vi "draw_points.vi"(8 "XY Graph Ref In":refnum<vi>, 9 "Cycle":string(combo), 10 "T cluster":T2, 11 "P cluster":T3) -> (2 "XY Graph Ref Out":refnum<vi>, 3 "Table":string[][](array[string]))   [LabVIEW 2017]
panel:
  out "points array":T1(array[cluster])
  out "error out":errorcluster
  out "Application Directory 2":path
  out "Application Directory":path
  out "Points":dbl[][](array[numeric])
  out "P10":dbl
  out "XY Graph":cluster{dbl[], dbl[]}(graph)
  out "output cluster":cluster{dbl[], dbl[]}
  out "P11":dbl
  out "P5":dbl
  out "P4":dbl
  out "P3":dbl
  out "P2":dbl
  out "P1":dbl
  out "T11":dbl
  out "T10":dbl
  out "T9":dbl
  out "T8":dbl
  out "T7":dbl
  out "T6":dbl
  out "T5":dbl
  out "T4":dbl
  out "T3":dbl
  out "T2":dbl
  out "T1":dbl
  out "H Point 3":dbl
  out "Loop Iteration":i32
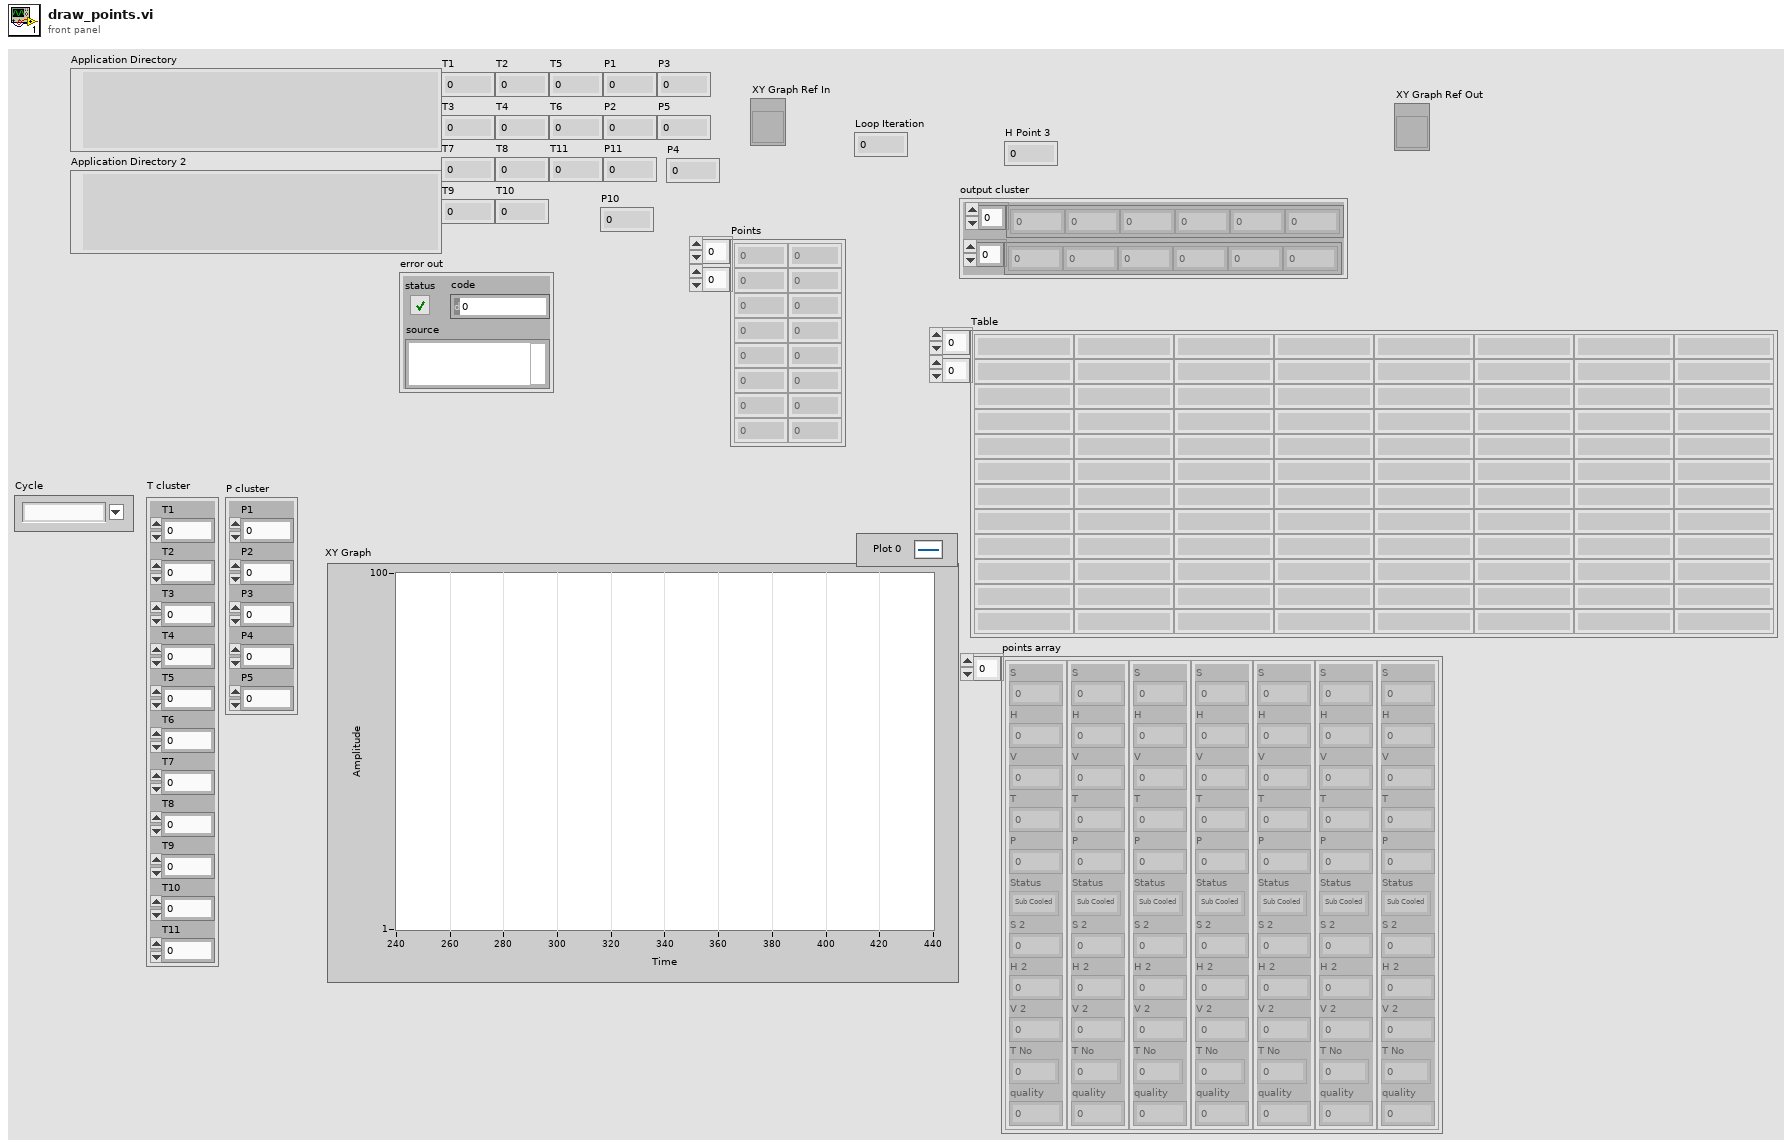
[diagram p1: front panel]
types:
  T1 = cluster{"S":dbl, "H":dbl, "V":dbl, "T":dbl, "P":dbl, "Status":enum16{"Sub Cooled", "Saturation", "Super Heated"}, "S 2":dbl, "H 2":dbl, "V 2":dbl, "T No":enum16{"0", "1", "2", "3", "4"}, "quality":dbl}[]
  T2 = cluster{"T1":dbl, "T2":dbl, "T3":dbl, "T4":dbl, "T5":dbl, "T6":dbl, "T7":dbl, "T8":dbl, "T9":dbl, "T10":dbl, "T11":dbl}
  T3 = cluster{"P1":dbl, "P2":dbl, "P3":dbl, "P4":dbl, "P5":dbl}
  T4 = cluster{"Name":string, "Color":u32, "Style":u8, "Point Style":u8, "Name Visible":bool, "Allow Drag":bool, "Annotation Mode":u32, "Plot":i32, "Index":i32, "Position":cluster{"X":dbl, "Y":dbl}, "X Scale":u32, "Y Scale":u32, "Show Arrow":bool, "Lock Name":bool, "Plot Area":i32, "Label Offset":cluster{"X":dbl, "Y":dbl}}
  T5 = cluster{"S":dbl, "H":dbl, "V":dbl, "T":dbl, "P":dbl, "Status":enum16{"Sub Cooled", "Saturation", "Super Heated"}, "S 2":dbl, "H 2":dbl, "V 2":dbl, "T No":enum16{"0", "1", "2", "3", "4"}, "quality":dbl}
  T6 = enum16{"Sub Cooled", "Saturation", "Super Heated"}
  T7 = typedef "LVAnnotationListTypeDef.ctl" = cluster{"Name":string, "Color":u32, "Style":u8, "Point Style":u8, "Name Visible":bool, "Allow Drag":bool, "Annotation Mode":u32, "Plot":i32, "Index":i32, "Position":cluster{"X":dbl, "Y":dbl}, "X Scale":u32, "Y Scale":u32, "Show Arrow":bool, "Lock Name":bool, "Plot Area":i32, "Label Offset":cluster{"X":dbl, "Y":dbl}}[]
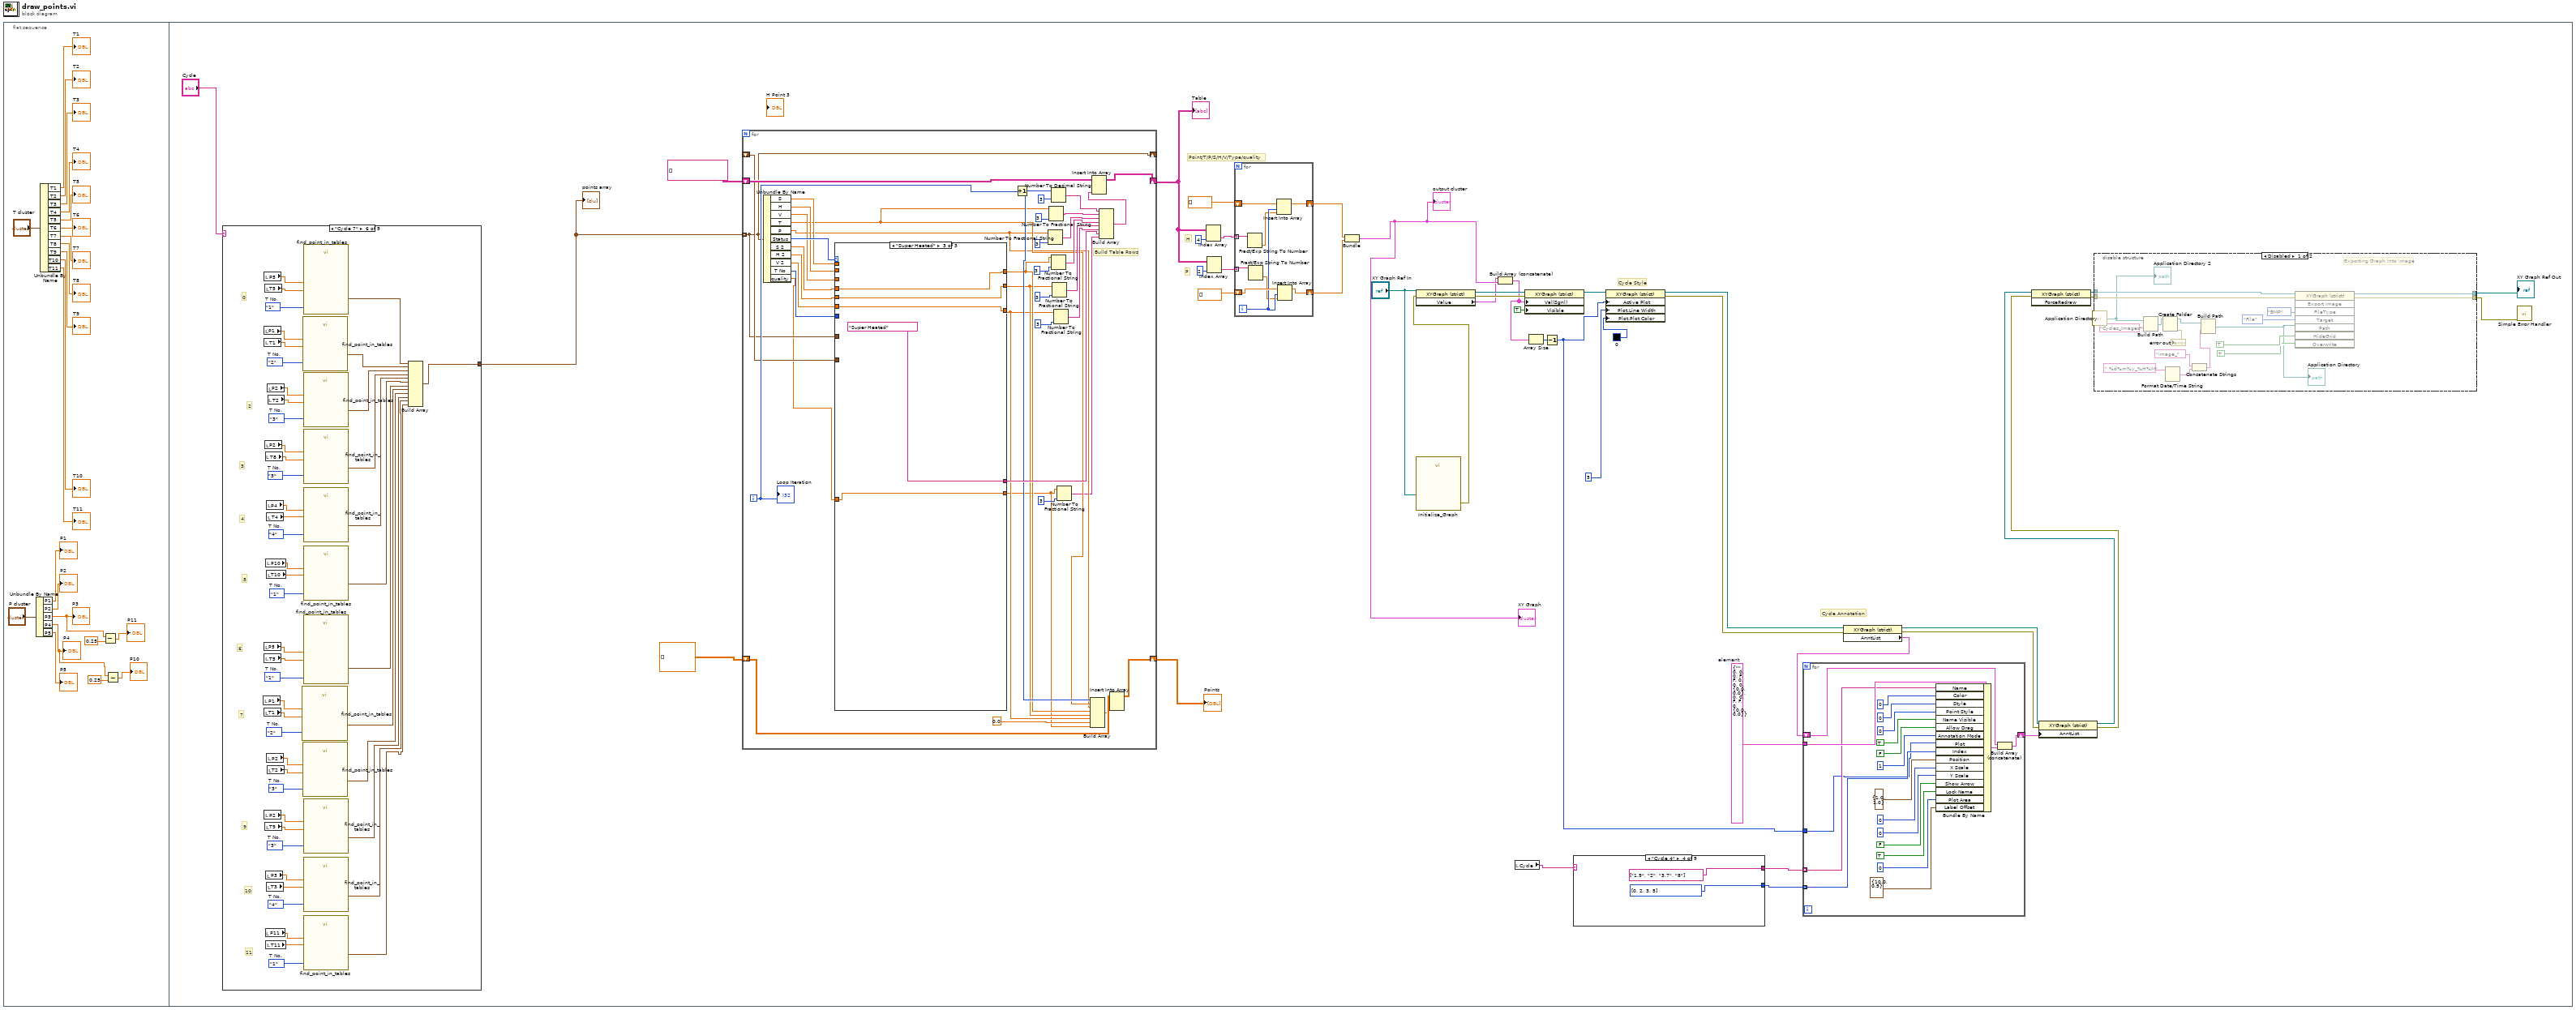
[diagram p0: block diagram]
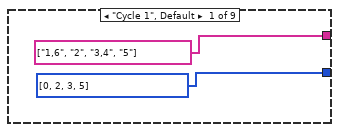
[diagram p3: hidden frame]
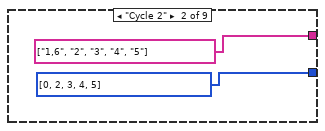
[diagram p4: hidden frame]
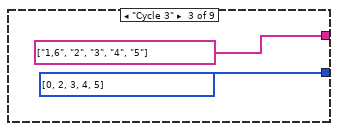
[diagram p5: hidden frame]
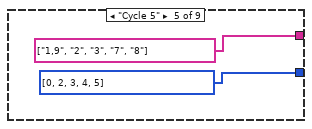
[diagram p6: hidden frame]
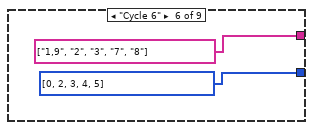
[diagram p7: hidden frame]
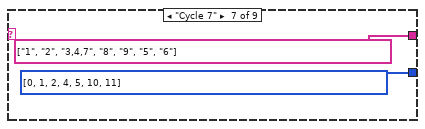
[diagram p8: hidden frame]
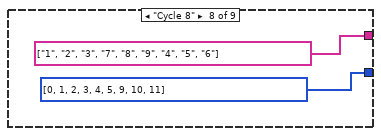
[diagram p9: hidden frame]
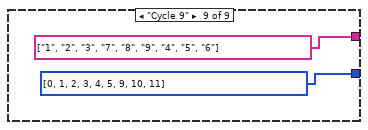
[diagram p10: hidden frame]
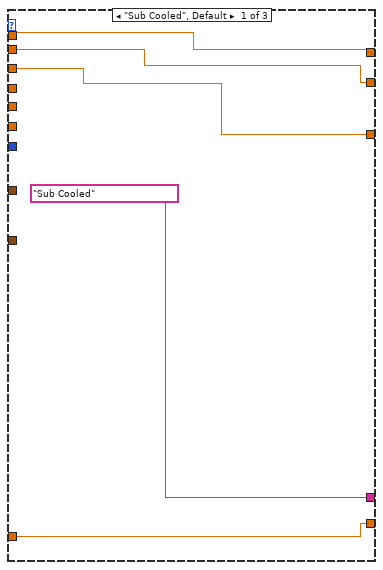
[diagram p11: hidden frame]
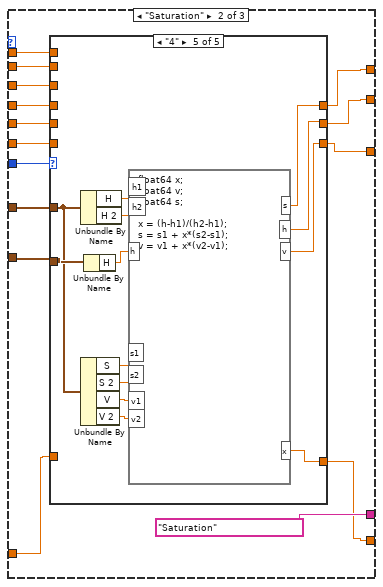
[diagram p12: hidden frame]
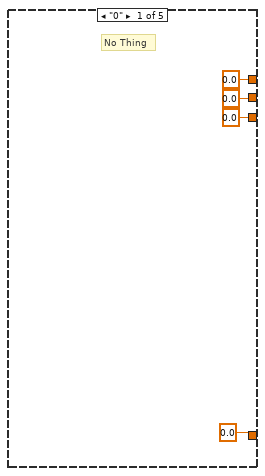
[diagram p13: hidden frame]
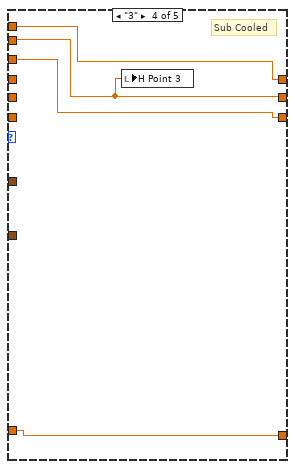
[diagram p16: hidden frame]
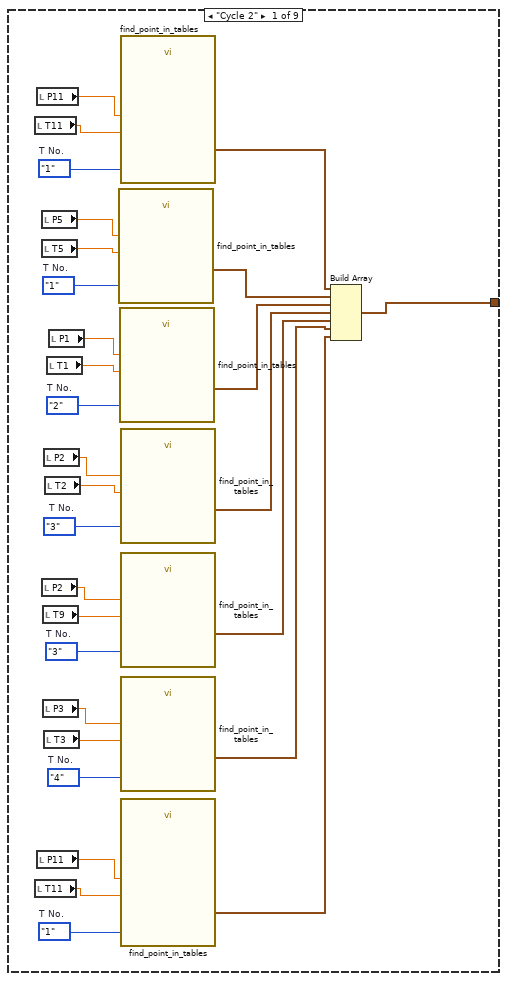
[diagram p17: hidden frame]
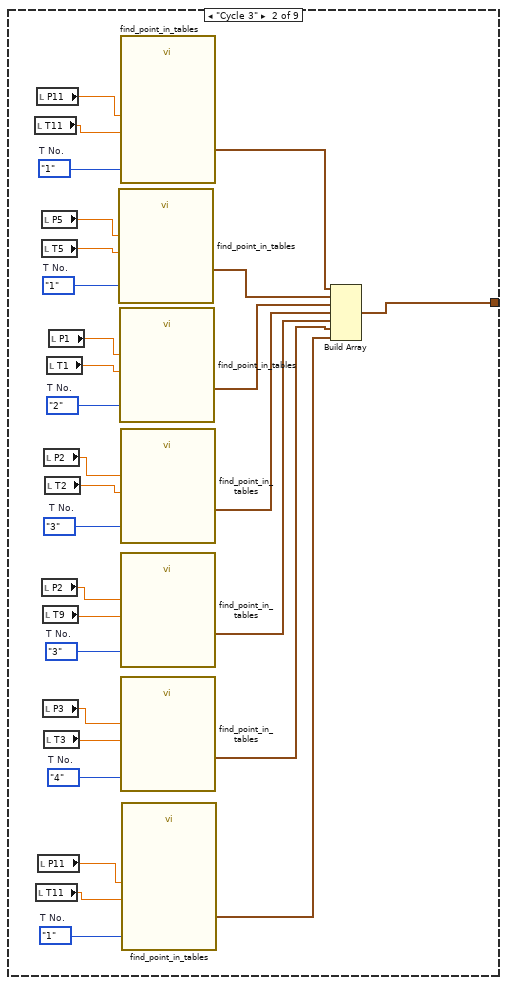
[diagram p18: hidden frame]
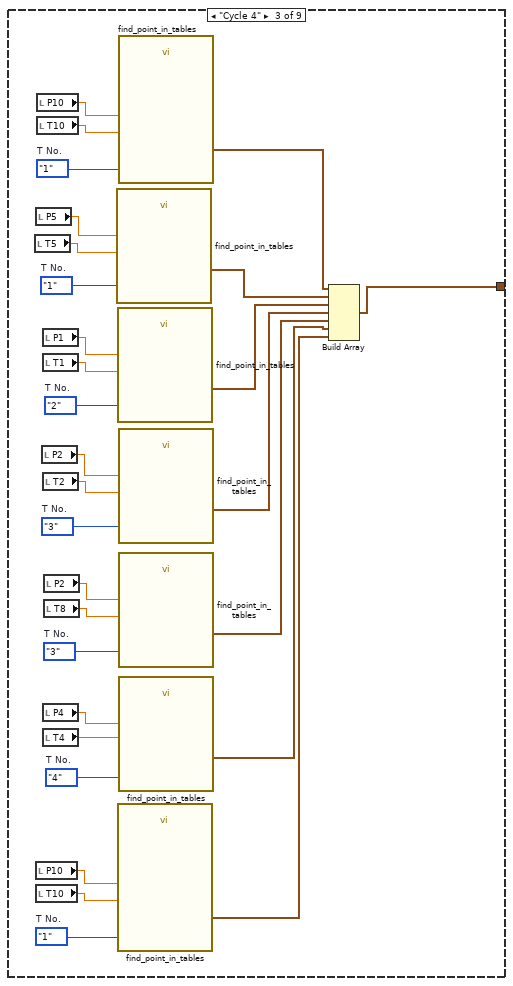
[diagram p19: hidden frame]
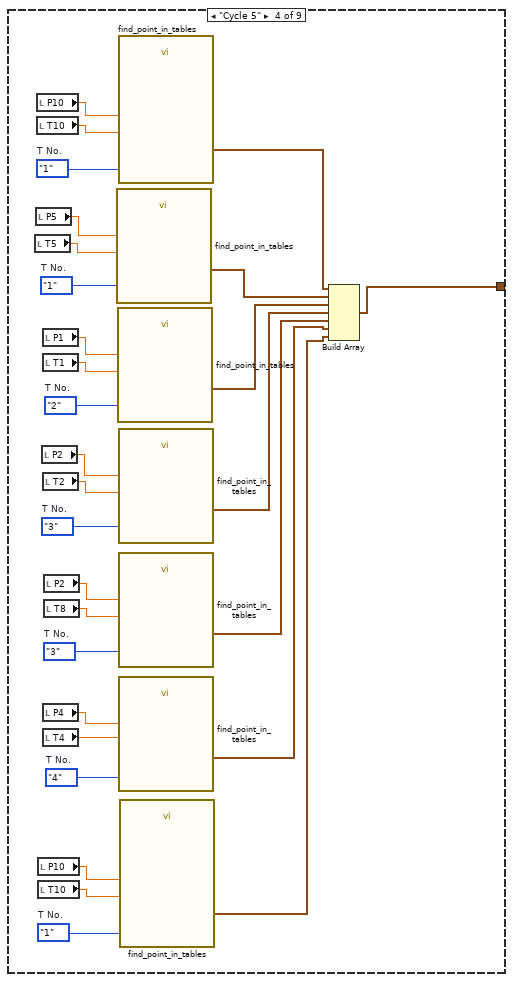
[diagram p20: hidden frame]
diagram:
  n1 = flat-sequence {
    frame #0 {
      n2 = Unbundle By Name("P cluster") -> ("P1"=→"P1":dbl, "P2"=→"P2":dbl, "P3"=w4:dbl, "P4"=w1:dbl, "P5"=→"P5":dbl)
      "P3" <- w4
      "P4" <- w1
      n3 = Unbundle By Name("T cluster") -> ("T1"=→"T1":dbl, "T2"=→"T2":dbl, "T3"=→"T3":dbl, "T4"=→"T4":dbl, "T5"=→"T5":dbl, "T6"=→"T6":dbl, "T7"=→"T7":dbl, "T8"=→"T8":dbl, "T9"=→"T9":dbl, "T10"=→"T10":dbl, "T11"=→"T11":dbl)
      n4 = Subtract(x=w4, y=0.25) -> (x-y=→"P11":dbl)
      n5 = Subtract(x=w1, y=0.25) -> (x-y=→"P10":dbl)
    }
    frame #1 {
      w41 = T4 {"Name"="", "Color"=0, "Style"=0, "Point Style"=0, "Name Visible"=FALSE, "Allow Drag"=FALSE, "Annotation Mode"=0, "Plot"=0, "Index"=0, "Position"={"X"=0.0, "Y"=0.0}, "X Scale"=0, "Y Scale"=0, "Show Arrow"=FALSE, "Lock Name"=FALSE, "Plot Area"=0, "Label Offset"={"X"=0.0, "Y"=0.0}}  # element
      # "Cycle Annotation"
      # "Cycle Style"
      # "H"
      # "P"
      # "Point/T/P/S/H/V/Type/quality"
      n6 = case shown="\"Cycle 7\"" "Cycle" {
        tunnel: [w232 w261 w302 w331 w360 w409 w458 w507 w540] -> w23
        frame "Cycle 2" {
          w229 = enum16{"0", "1", "2", "3", "4"}."1"  # T No.
          w245 = enum16{"0", "1", "2", "3", "4"}."4"  # T No.
          w246 = enum16{"0", "1", "2", "3", "4"}."3"  # T No.
          w247 = enum16{"0", "1", "2", "3", "4"}."3"  # T No.
          w248 = enum16{"0", "1", "2", "3", "4"}."2"  # T No.
          w249 = enum16{"0", "1", "2", "3", "4"}."1"  # T No.
          w250 = enum16{"0", "1", "2", "3", "4"}."1"  # T No.
          n7 = local read "T11"() -> (w243:dbl)
          n8 = local read "T11"() -> (w231:dbl)
          n9 = local read "P11"() -> (w244:dbl)
          n10 = local read "P11"() -> (w230:dbl)
          n11 = local read "P5"() -> (w242:dbl)
          n12 = local read "T5"() -> (w241:dbl)
          n13 = local read "P2"() -> (w236:dbl)
          n14 = local read "T9"() -> (w235:dbl)
          n15 = local read "P3"() -> (w234:dbl)
          n16 = local read "P2"() -> (w238:dbl)
          n17 = local read "T3"() -> (w233:dbl)
          n18 = local read "T2"() -> (w237:dbl)
          n19 = local read "T1"() -> (w239:dbl)
          n20 = local read "P1"() -> (w240:dbl)
          n21 = call "find_point_in_tables.vi"("T No."=w249, "T Search"=w241, "P Search"=w242) -> ("Point"=w254:T5)  [unwired: 7 in]
          n22 = call "find_point_in_tables.vi"("T No."=w248, "T Search"=w239, "P Search"=w240) -> ("Point"=w255:T5)  [unwired: 7 in]
          n23 = call "find_point_in_tables.vi"("T No."=w250, "T Search"=w243, "P Search"=w244) -> ("Point"=w253:T5)  [unwired: 7 in]
          n24 = call "find_point_in_tables.vi"("T No."=w247, "T Search"=w237, "P Search"=w238) -> ("Point"=w256:T5)  [unwired: 7 in]
          n25 = call "find_point_in_tables.vi"("T No."=w246, "T Search"=w235, "P Search"=w236) -> ("Point"=w252:T5)  [unwired: 7 in]
          n26 = call "find_point_in_tables.vi"("T No."=w245, "T Search"=w233, "P Search"=w234) -> ("Point"=w251:T5)  [unwired: 7 in]
          n27 = call "find_point_in_tables.vi"("T No."=w229, "T Search"=w231, "P Search"=w230) -> ("Point"=w228:T5)  [unwired: 7 in]
          n28 = Build Array(w253, w254, w255, w256, w252, w251, w228) -> (w232:T1)
        }
        frame "Cycle 3" {
          w258 = enum16{"0", "1", "2", "3", "4"}."1"  # T No.
          w274 = enum16{"0", "1", "2", "3", "4"}."4"  # T No.
          w275 = enum16{"0", "1", "2", "3", "4"}."3"  # T No.
          w276 = enum16{"0", "1", "2", "3", "4"}."3"  # T No.
          w277 = enum16{"0", "1", "2", "3", "4"}."2"  # T No.
          w278 = enum16{"0", "1", "2", "3", "4"}."1"  # T No.
          w279 = enum16{"0", "1", "2", "3", "4"}."1"  # T No.
          n29 = local read "T11"() -> (w272:dbl)
          n30 = local read "T11"() -> (w260:dbl)
          n31 = local read "P11"() -> (w273:dbl)
          n32 = local read "P11"() -> (w259:dbl)
          n33 = local read "P5"() -> (w271:dbl)
          n34 = local read "T5"() -> (w270:dbl)
          n35 = local read "P2"() -> (w265:dbl)
          n36 = local read "T9"() -> (w264:dbl)
          n37 = local read "P3"() -> (w263:dbl)
          n38 = local read "P2"() -> (w267:dbl)
          n39 = local read "T3"() -> (w262:dbl)
          n40 = local read "T2"() -> (w266:dbl)
          n41 = local read "T1"() -> (w268:dbl)
          n42 = local read "P1"() -> (w269:dbl)
          n43 = call "find_point_in_tables.vi"("T No."=w278, "T Search"=w270, "P Search"=w271) -> ("Point"=w283:T5)  [unwired: 7 in]
          n44 = call "find_point_in_tables.vi"("T No."=w277, "T Search"=w268, "P Search"=w269) -> ("Point"=w284:T5)  [unwired: 7 in]
          n45 = call "find_point_in_tables.vi"("T No."=w279, "T Search"=w272, "P Search"=w273) -> ("Point"=w282:T5)  [unwired: 7 in]
          n46 = call "find_point_in_tables.vi"("T No."=w276, "T Search"=w266, "P Search"=w267) -> ("Point"=w285:T5)  [unwired: 7 in]
          n47 = call "find_point_in_tables.vi"("T No."=w275, "T Search"=w264, "P Search"=w265) -> ("Point"=w281:T5)  [unwired: 7 in]
          n48 = call "find_point_in_tables.vi"("T No."=w274, "T Search"=w262, "P Search"=w263) -> ("Point"=w280:T5)  [unwired: 7 in]
          n49 = call "find_point_in_tables.vi"("T No."=w258, "T Search"=w260, "P Search"=w259) -> ("Point"=w257:T5)  [unwired: 7 in]
          n50 = Build Array(w282, w283, w284, w285, w281, w280, w257) -> (w261:T1)
        }
        frame "Cycle 4" {
          w287 = enum16{"0", "1", "2", "3", "4"}."1"  # T No.
          w303 = enum16{"0", "1", "2", "3", "4"}."4"  # T No.
          w304 = enum16{"0", "1", "2", "3", "4"}."3"  # T No.
          w305 = enum16{"0", "1", "2", "3", "4"}."3"  # T No.
          w306 = enum16{"0", "1", "2", "3", "4"}."2"  # T No.
          w307 = enum16{"0", "1", "2", "3", "4"}."1"  # T No.
          w308 = enum16{"0", "1", "2", "3", "4"}."1"  # T No.
          n51 = local read "T5"() -> (w298:dbl)
          n52 = local read "P5"() -> (w299:dbl)
          n53 = local read "P10"() -> (w289:dbl)
          n54 = local read "T10"() -> (w288:dbl)
          n55 = local read "P10"() -> (w300:dbl)
          n56 = local read "T10"() -> (w301:dbl)
          n57 = local read "P2"() -> (w295:dbl)
          n58 = local read "P1"() -> (w297:dbl)
          n59 = local read "T1"() -> (w296:dbl)
          n60 = local read "T2"() -> (w294:dbl)
          n61 = local read "P4"() -> (w291:dbl)
          n62 = local read "T4"() -> (w290:dbl)
          n63 = local read "P2"() -> (w293:dbl)
          n64 = local read "T8"() -> (w292:dbl)
          n65 = call "find_point_in_tables.vi"("T No."=w307, "T Search"=w298, "P Search"=w299) -> ("Point"=w312:T5)  [unwired: 7 in]
          n66 = call "find_point_in_tables.vi"("T No."=w306, "T Search"=w296, "P Search"=w297) -> ("Point"=w313:T5)  [unwired: 7 in]
          n67 = call "find_point_in_tables.vi"("T No."=w287, "T Search"=w288, "P Search"=w289) -> ("Point"=w286:T5)  [unwired: 7 in]
          n68 = call "find_point_in_tables.vi"("T No."=w308, "T Search"=w301, "P Search"=w300) -> ("Point"=w311:T5)  [unwired: 7 in]
          n69 = call "find_point_in_tables.vi"("T No."=w305, "T Search"=w294, "P Search"=w295) -> ("Point"=w314:T5)  [unwired: 7 in]
          n70 = call "find_point_in_tables.vi"("T No."=w304, "T Search"=w292, "P Search"=w293) -> ("Point"=w310:T5)  [unwired: 7 in]
          n71 = call "find_point_in_tables.vi"("T No."=w303, "T Search"=w290, "P Search"=w291) -> ("Point"=w309:T5)  [unwired: 7 in]
          n72 = Build Array(w311, w312, w313, w314, w310, w309, w286) -> (w302:T1)
        }
        frame "Cycle 5" {
          w316 = enum16{"0", "1", "2", "3", "4"}."1"  # T No.
          w332 = enum16{"0", "1", "2", "3", "4"}."4"  # T No.
          w333 = enum16{"0", "1", "2", "3", "4"}."3"  # T No.
          w334 = enum16{"0", "1", "2", "3", "4"}."3"  # T No.
          w335 = enum16{"0", "1", "2", "3", "4"}."2"  # T No.
          w336 = enum16{"0", "1", "2", "3", "4"}."1"  # T No.
          w337 = enum16{"0", "1", "2", "3", "4"}."1"  # T No.
          n73 = local read "T5"() -> (w327:dbl)
          n74 = local read "P5"() -> (w328:dbl)
          n75 = local read "P10"() -> (w329:dbl)
          n76 = local read "T10"() -> (w330:dbl)
          n77 = local read "P10"() -> (w318:dbl)
          n78 = local read "T10"() -> (w317:dbl)
          n79 = local read "P2"() -> (w324:dbl)
          n80 = local read "P1"() -> (w326:dbl)
          n81 = local read "T1"() -> (w325:dbl)
          n82 = local read "T2"() -> (w323:dbl)
          n83 = local read "P4"() -> (w320:dbl)
          n84 = local read "T4"() -> (w319:dbl)
          n85 = local read "P2"() -> (w322:dbl)
          n86 = local read "T8"() -> (w321:dbl)
          n87 = call "find_point_in_tables.vi"("T No."=w336, "T Search"=w327, "P Search"=w328) -> ("Point"=w341:T5)  [unwired: 7 in]
          n88 = call "find_point_in_tables.vi"("T No."=w335, "T Search"=w325, "P Search"=w326) -> ("Point"=w342:T5)  [unwired: 7 in]
          n89 = call "find_point_in_tables.vi"("T No."=w337, "T Search"=w330, "P Search"=w329) -> ("Point"=w340:T5)  [unwired: 7 in]
          n90 = call "find_point_in_tables.vi"("T No."=w334, "T Search"=w323, "P Search"=w324) -> ("Point"=w343:T5)  [unwired: 7 in]
          n91 = call "find_point_in_tables.vi"("T No."=w333, "T Search"=w321, "P Search"=w322) -> ("Point"=w339:T5)  [unwired: 7 in]
          n92 = call "find_point_in_tables.vi"("T No."=w332, "T Search"=w319, "P Search"=w320) -> ("Point"=w338:T5)  [unwired: 7 in]
          n93 = call "find_point_in_tables.vi"("T No."=w316, "T Search"=w317, "P Search"=w318) -> ("Point"=w315:T5)  [unwired: 7 in]
          n94 = Build Array(w340, w341, w342, w343, w339, w338, w315) -> (w331:T1)
        }
        frame "Cycle 6" {
          w345 = enum16{"0", "1", "2", "3", "4"}."1"  # T No.
          w361 = enum16{"0", "1", "2", "3", "4"}."4"  # T No.
          w362 = enum16{"0", "1", "2", "3", "4"}."3"  # T No.
          w363 = enum16{"0", "1", "2", "3", "4"}."3"  # T No.
          w364 = enum16{"0", "1", "2", "3", "4"}."2"  # T No.
          w365 = enum16{"0", "1", "2", "3", "4"}."1"  # T No.
          w366 = enum16{"0", "1", "2", "3", "4"}."1"  # T No.
          n95 = local read "T5"() -> (w356:dbl)
          n96 = local read "P5"() -> (w357:dbl)
          n97 = local read "P10"() -> (w358:dbl)
          n98 = local read "T10"() -> (w359:dbl)
          n99 = local read "P10"() -> (w347:dbl)
          n100 = local read "T10"() -> (w346:dbl)
          n101 = local read "P2"() -> (w353:dbl)
          n102 = local read "P1"() -> (w355:dbl)
          n103 = local read "T1"() -> (w354:dbl)
          n104 = local read "T2"() -> (w352:dbl)
          n105 = local read "P4"() -> (w349:dbl)
          n106 = local read "T4"() -> (w348:dbl)
          n107 = local read "P2"() -> (w351:dbl)
          n108 = local read "T8"() -> (w350:dbl)
          n109 = call "find_point_in_tables.vi"("T No."=w365, "T Search"=w356, "P Search"=w357) -> ("Point"=w370:T5)  [unwired: 7 in]
          n110 = call "find_point_in_tables.vi"("T No."=w364, "T Search"=w354, "P Search"=w355) -> ("Point"=w371:T5)  [unwired: 7 in]
          n111 = call "find_point_in_tables.vi"("T No."=w366, "T Search"=w359, "P Search"=w358) -> ("Point"=w369:T5)  [unwired: 7 in]
          n112 = call "find_point_in_tables.vi"("T No."=w363, "T Search"=w352, "P Search"=w353) -> ("Point"=w372:T5)  [unwired: 7 in]
          n113 = call "find_point_in_tables.vi"("T No."=w362, "T Search"=w350, "P Search"=w351) -> ("Point"=w368:T5)  [unwired: 7 in]
          n114 = call "find_point_in_tables.vi"("T No."=w361, "T Search"=w348, "P Search"=w349) -> ("Point"=w367:T5)  [unwired: 7 in]
          n115 = call "find_point_in_tables.vi"("T No."=w345, "T Search"=w346, "P Search"=w347) -> ("Point"=w344:T5)  [unwired: 7 in]
          n116 = Build Array(w369, w370, w371, w372, w368, w367, w344) -> (w360:T1)
        }
        frame "Cycle 7" {
          w384 = enum16{"0", "1", "2", "3", "4"}."1"  # T No.
          w383 = enum16{"0", "1", "2", "3", "4"}."4"  # T No.
          w382 = enum16{"0", "1", "2", "3", "4"}."3"  # T No.
          w381 = enum16{"0", "1", "2", "3", "4"}."3"  # T No.
          w380 = enum16{"0", "1", "2", "3", "4"}."2"  # T No.
          w379 = enum16{"0", "1", "2", "3", "4"}."1"  # T No.
          w410 = enum16{"0", "1", "2", "3", "4"}."1"  # T No.
          w411 = enum16{"0", "1", "2", "3", "4"}."4"  # T No.
          w412 = enum16{"0", "1", "2", "3", "4"}."3"  # T No.
          w413 = enum16{"0", "1", "2", "3", "4"}."3"  # T No.
          w414 = enum16{"0", "1", "2", "3", "4"}."2"  # T No.
          w415 = enum16{"0", "1", "2", "3", "4"}."1"  # T No.
          # "11"
          # "10"
          # "9"
          # "8"
          # "7"
          # "6"
          # "5"
          # "4"
          # "3"
          # "2"
          # "1"
          # "0"
          n117 = local read "P1"() -> (w387:dbl)
          n118 = local read "P1"() -> (w406:dbl)
          n119 = local read "P5"() -> (w385:dbl)
          n120 = local read "T1"() -> (w388:dbl)
          n121 = local read "P5"() -> (w408:dbl)
          n122 = local read "T1"() -> (w405:dbl)
          n123 = local read "T5"() -> (w386:dbl)
          n124 = local read "P2"() -> (w391:dbl)
          n125 = local read "T5"() -> (w407:dbl)
          n126 = local read "P2"() -> (w402:dbl)
          n127 = local read "T9"() -> (w392:dbl)
          n128 = local read "T8"() -> (w401:dbl)
          n129 = local read "P11"() -> (w395:dbl)
          n130 = local read "P10"() -> (w398:dbl)
          n131 = local read "P3"() -> (w393:dbl)
          n132 = local read "T11"() -> (w396:dbl)
          n133 = local read "P4"() -> (w400:dbl)
          n134 = local read "T10"() -> (w397:dbl)
          n135 = local read "T3"() -> (w394:dbl)
          n136 = local read "T4"() -> (w399:dbl)
          n137 = local read "P2"() -> (w389:dbl)
          n138 = local read "P2"() -> (w404:dbl)
          n139 = local read "T2"() -> (w390:dbl)
          n140 = local read "T2"() -> (w403:dbl)
          n141 = call "find_point_in_tables.vi"("T No."=w380, "T Search"=w388, "P Search"=w387) -> ("Point"=w377:T5)  [unwired: 7 in]
          n142 = call "find_point_in_tables.vi"("T No."=w414, "T Search"=w405, "P Search"=w406) -> ("Point"=w419:T5)  [unwired: 7 in]
          n143 = call "find_point_in_tables.vi"("T No."=w381, "T Search"=w390, "P Search"=w389) -> ("Point"=w376:T5)  [unwired: 7 in]
          n144 = call "find_point_in_tables.vi"("T No."=w413, "T Search"=w403, "P Search"=w404) -> ("Point"=w420:T5)  [unwired: 7 in]
          n145 = call "find_point_in_tables.vi"("T No."=w379, "T Search"=w386, "P Search"=w385) -> ("Point"=w378:T5)  [unwired: 7 in]
          n146 = call "find_point_in_tables.vi"("T No."=w382, "T Search"=w392, "P Search"=w391) -> ("Point"=w375:T5)  [unwired: 7 in]
          n147 = call "find_point_in_tables.vi"("T No."=w383, "T Search"=w394, "P Search"=w393) -> ("Point"=w374:T5)  [unwired: 7 in]
          n148 = call "find_point_in_tables.vi"("T No."=w384, "T Search"=w396, "P Search"=w395) -> ("Point"=w373:T5)  [unwired: 7 in]
          n149 = call "find_point_in_tables.vi"("T No."=w415, "T Search"=w407, "P Search"=w408) -> ("Point"=w418:T5)  [unwired: 7 in]
          n150 = call "find_point_in_tables.vi"("T No."=w412, "T Search"=w401, "P Search"=w402) -> ("Point"=w421:T5)  [unwired: 7 in]
          n151 = call "find_point_in_tables.vi"("T No."=w411, "T Search"=w399, "P Search"=w400) -> ("Point"=w417:T5)  [unwired: 7 in]
          n152 = call "find_point_in_tables.vi"("T No."=w410, "T Search"=w397, "P Search"=w398) -> ("Point"=w416:T5)  [unwired: 7 in]
          n153 = Build Array(w418, w419, w420, w421, w417, w416, w378, w377, w376, w375, w374, w373) -> (w409:T1)
        }
        frame "Cycle 8" {
          w433 = enum16{"0", "1", "2", "3", "4"}."1"  # T No.
          w432 = enum16{"0", "1", "2", "3", "4"}."4"  # T No.
          w431 = enum16{"0", "1", "2", "3", "4"}."3"  # T No.
          w430 = enum16{"0", "1", "2", "3", "4"}."3"  # T No.
          w429 = enum16{"0", "1", "2", "3", "4"}."2"  # T No.
          w428 = enum16{"0", "1", "2", "3", "4"}."1"  # T No.
          w459 = enum16{"0", "1", "2", "3", "4"}."1"  # T No.
          w460 = enum16{"0", "1", "2", "3", "4"}."4"  # T No.
          w461 = enum16{"0", "1", "2", "3", "4"}."3"  # T No.
          w462 = enum16{"0", "1", "2", "3", "4"}."3"  # T No.
          w463 = enum16{"0", "1", "2", "3", "4"}."2"  # T No.
          w464 = enum16{"0", "1", "2", "3", "4"}."1"  # T No.
          n154 = local read "P1"() -> (w436:dbl)
          n155 = local read "P1"() -> (w455:dbl)
          n156 = local read "P5"() -> (w434:dbl)
          n157 = local read "T1"() -> (w437:dbl)
          n158 = local read "P5"() -> (w457:dbl)
          n159 = local read "T1"() -> (w454:dbl)
          n160 = local read "T5"() -> (w435:dbl)
          n161 = local read "P2"() -> (w440:dbl)
          n162 = local read "T5"() -> (w456:dbl)
          n163 = local read "P2"() -> (w451:dbl)
          n164 = local read "T9"() -> (w441:dbl)
          n165 = local read "T8"() -> (w450:dbl)
          n166 = local read "P11"() -> (w444:dbl)
          n167 = local read "P10"() -> (w447:dbl)
          n168 = local read "P3"() -> (w442:dbl)
          n169 = local read "T11"() -> (w445:dbl)
          n170 = local read "P4"() -> (w449:dbl)
          n171 = local read "T10"() -> (w446:dbl)
          n172 = local read "T3"() -> (w443:dbl)
          n173 = local read "T4"() -> (w448:dbl)
          n174 = local read "T2"() -> (w438:dbl)
          n175 = local read "P2"() -> (w453:dbl)
          n176 = local read "P2"() -> (w439:dbl)
          n177 = local read "T2"() -> (w452:dbl)
          n178 = call "find_point_in_tables.vi"("T No."=w429, "T Search"=w437, "P Search"=w436) -> ("Point"=w426:T5)  [unwired: 7 in]
          n179 = call "find_point_in_tables.vi"("T No."=w463, "T Search"=w454, "P Search"=w455) -> ("Point"=w468:T5)  [unwired: 7 in]
          n180 = call "find_point_in_tables.vi"("T No."=w430, "T Search"=w439, "P Search"=w438) -> ("Point"=w425:T5)  [unwired: 7 in]
          n181 = call "find_point_in_tables.vi"("T No."=w462, "T Search"=w452, "P Search"=w453) -> ("Point"=w469:T5)  [unwired: 7 in]
          n182 = call "find_point_in_tables.vi"("T No."=w428, "T Search"=w435, "P Search"=w434) -> ("Point"=w427:T5)  [unwired: 7 in]
          n183 = call "find_point_in_tables.vi"("T No."=w431, "T Search"=w441, "P Search"=w440) -> ("Point"=w424:T5)  [unwired: 7 in]
          n184 = call "find_point_in_tables.vi"("T No."=w432, "T Search"=w443, "P Search"=w442) -> ("Point"=w423:T5)  [unwired: 7 in]
          n185 = call "find_point_in_tables.vi"("T No."=w433, "T Search"=w445, "P Search"=w444) -> ("Point"=w422:T5)  [unwired: 7 in]
          n186 = call "find_point_in_tables.vi"("T No."=w464, "T Search"=w456, "P Search"=w457) -> ("Point"=w467:T5)  [unwired: 7 in]
          n187 = call "find_point_in_tables.vi"("T No."=w461, "T Search"=w450, "P Search"=w451) -> ("Point"=w470:T5)  [unwired: 7 in]
          n188 = call "find_point_in_tables.vi"("T No."=w460, "T Search"=w448, "P Search"=w449) -> ("Point"=w466:T5)  [unwired: 7 in]
          n189 = call "find_point_in_tables.vi"("T No."=w459, "T Search"=w446, "P Search"=w447) -> ("Point"=w465:T5)  [unwired: 7 in]
          n190 = Build Array(w467, w468, w469, w470, w466, w465, w427, w426, w425, w424, w423, w422) -> (w458:T1)
        }
        frame "Cycle 9" {
          w482 = enum16{"0", "1", "2", "3", "4"}."1"  # T No.
          w481 = enum16{"0", "1", "2", "3", "4"}."4"  # T No.
          w480 = enum16{"0", "1", "2", "3", "4"}."3"  # T No.
          w479 = enum16{"0", "1", "2", "3", "4"}."3"  # T No.
          w478 = enum16{"0", "1", "2", "3", "4"}."2"  # T No.
          w477 = enum16{"0", "1", "2", "3", "4"}."1"  # T No.
          w508 = enum16{"0", "1", "2", "3", "4"}."1"  # T No.
          w509 = enum16{"0", "1", "2", "3", "4"}."4"  # T No.
          w510 = enum16{"0", "1", "2", "3", "4"}."3"  # T No.
          w511 = enum16{"0", "1", "2", "3", "4"}."3"  # T No.
          w512 = enum16{"0", "1", "2", "3", "4"}."2"  # T No.
          w513 = enum16{"0", "1", "2", "3", "4"}."1"  # T No.
          n191 = local read "P1"() -> (w485:dbl)
          n192 = local read "P1"() -> (w504:dbl)
          n193 = local read "P5"() -> (w483:dbl)
          n194 = local read "T1"() -> (w486:dbl)
          n195 = local read "P5"() -> (w506:dbl)
          n196 = local read "T1"() -> (w503:dbl)
          n197 = local read "T5"() -> (w484:dbl)
          n198 = local read "P2"() -> (w489:dbl)
          n199 = local read "T5"() -> (w505:dbl)
          n200 = local read "P2"() -> (w500:dbl)
          n201 = local read "T9"() -> (w490:dbl)
          n202 = local read "T8"() -> (w499:dbl)
          n203 = local read "P11"() -> (w493:dbl)
          n204 = local read "P10"() -> (w496:dbl)
          n205 = local read "P3"() -> (w491:dbl)
          n206 = local read "T11"() -> (w494:dbl)
          n207 = local read "P4"() -> (w498:dbl)
          n208 = local read "T10"() -> (w495:dbl)
          n209 = local read "T3"() -> (w492:dbl)
          n210 = local read "T4"() -> (w497:dbl)
          n211 = local read "T2"() -> (w487:dbl)
          n212 = local read "P2"() -> (w502:dbl)
          n213 = local read "P2"() -> (w488:dbl)
          n214 = local read "T2"() -> (w501:dbl)
          n215 = call "find_point_in_tables.vi"("T No."=w478, "T Search"=w486, "P Search"=w485) -> ("Point"=w475:T5)  [unwired: 7 in]
          n216 = call "find_point_in_tables.vi"("T No."=w512, "T Search"=w503, "P Search"=w504) -> ("Point"=w517:T5)  [unwired: 7 in]
          n217 = call "find_point_in_tables.vi"("T No."=w479, "T Search"=w488, "P Search"=w487) -> ("Point"=w474:T5)  [unwired: 7 in]
          n218 = call "find_point_in_tables.vi"("T No."=w511, "T Search"=w501, "P Search"=w502) -> ("Point"=w518:T5)  [unwired: 7 in]
          n219 = call "find_point_in_tables.vi"("T No."=w477, "T Search"=w484, "P Search"=w483) -> ("Point"=w476:T5)  [unwired: 7 in]
          n220 = call "find_point_in_tables.vi"("T No."=w480, "T Search"=w490, "P Search"=w489) -> ("Point"=w473:T5)  [unwired: 7 in]
          n221 = call "find_point_in_tables.vi"("T No."=w481, "T Search"=w492, "P Search"=w491) -> ("Point"=w472:T5)  [unwired: 7 in]
          n222 = call "find_point_in_tables.vi"("T No."=w482, "T Search"=w494, "P Search"=w493) -> ("Point"=w471:T5)  [unwired: 7 in]
          n223 = call "find_point_in_tables.vi"("T No."=w513, "T Search"=w505, "P Search"=w506) -> ("Point"=w516:T5)  [unwired: 7 in]
          n224 = call "find_point_in_tables.vi"("T No."=w510, "T Search"=w499, "P Search"=w500) -> ("Point"=w519:T5)  [unwired: 7 in]
          n225 = call "find_point_in_tables.vi"("T No."=w509, "T Search"=w497, "P Search"=w498) -> ("Point"=w515:T5)  [unwired: 7 in]
          n226 = call "find_point_in_tables.vi"("T No."=w508, "T Search"=w495, "P Search"=w496) -> ("Point"=w514:T5)  [unwired: 7 in]
          n227 = Build Array(w516, w517, w518, w519, w515, w514, w476, w475, w474, w473, w472, w471) -> (w507:T1)
        }
        frame "Cycle 1", Default {
          w521 = enum16{"0", "1", "2", "3", "4"}."1"  # T No.
          w538 = enum16{"0", "1", "2", "3", "4"}."4"  # T No.
          w539 = enum16{"0", "1", "2", "3", "4"}."3"  # T No.
          w544 = enum16{"0", "1", "2", "3", "4"}."3"  # T No.
          w543 = enum16{"0", "1", "2", "3", "4"}."2"  # T No.
          w542 = enum16{"0", "1", "2", "3", "4"}."1"  # T No.
          w541 = enum16{"0", "1", "2", "3", "4"}."1"  # T No.
          n228 = local read "P11"() -> (w535:dbl)
          n229 = local read "T11"() -> (w534:dbl)
          n230 = local read "P11"() -> (w522:dbl)
          n231 = local read "T11"() -> (w523:dbl)
          n232 = local read "P5"() -> (w533:dbl)
          n233 = local read "T5"() -> (w532:dbl)
          n234 = local read "P2"() -> (w529:dbl)
          n235 = local read "T2"() -> (w528:dbl)
          n236 = local read "P2"() -> (w527:dbl)
          n237 = local read "T9"() -> (w526:dbl)
          n238 = local read "P1"() -> (w531:dbl)
          n239 = local read "T1"() -> (w530:dbl)
          n240 = local read "P3"() -> (w525:dbl)
          n241 = local read "T3"() -> (w524:dbl)
          n242 = call "find_point_in_tables.vi"("T No."=w542, "T Search"=w532, "P Search"=w533) -> ("Point"=w546:T5)  [unwired: 7 in]
          n243 = call "find_point_in_tables.vi"("T No."=w543, "T Search"=w530, "P Search"=w531) -> ("Point"=w547:T5)  [unwired: 7 in]
          n244 = call "find_point_in_tables.vi"("T No."=w541, "T Search"=w534, "P Search"=w535) -> ("Point"=w545:T5)  [unwired: 7 in]
          n245 = call "find_point_in_tables.vi"("T No."=w544, "T Search"=w528, "P Search"=w529) -> ("Point"=w548:T5)  [unwired: 7 in]
          n246 = call "find_point_in_tables.vi"("T No."=w539, "T Search"=w526, "P Search"=w527) -> ("Point"=w537:T5)  [unwired: 7 in]
          n247 = call "find_point_in_tables.vi"("T No."=w538, "T Search"=w524, "P Search"=w525) -> ("Point"=w536:T5)  [unwired: 7 in]
          n248 = call "find_point_in_tables.vi"("T No."=w521, "T Search"=w523, "P Search"=w522) -> ("Point"=w520:T5)  [unwired: 7 in]
          n249 = Build Array(w545, w546, w547, w548, w537, w536, w520) -> (w540:T1)
        }
      }
      "points array" <- w23
      n250 = for {
        shift-right: [w171] -> w59
        shift-left: string[][] [] ("Table") -> [w172]
        tunnel: w23 -> [w138] mode=indexing
        shift-right: [w148] -> w48
        shift-left: dbl[][] [] -> [w147]
        shift-right: [w138] -> _
        shift-left: _ -> [w139]
        i -> [w149]
        # "Build Table Rows"
        n251 = Unbundle By Name(w138) -> ("S"=w167:dbl, "H"=w166:dbl, "V"=w165:dbl, "T"=w144:dbl, "P"=w143:dbl, "Status"=w170:T6, "S 2"=w164:dbl, "H 2"=w163:dbl, "V 2"=w162:dbl, "T No"=w160:enum16{"0", "1", "2", "3", "4"}, "quality"=w137:dbl)
        n252 = case shown="\"Super Heated\"" w170 {
          tunnel: ["Sub Cooled" "Saturation" "Super Heated"] -> w161
          tunnel: w167 -> [w177 w185 _]
          tunnel: w166 -> [w176 w184 _]
          tunnel: w165 -> [w175 w183 _]
          tunnel: w164 -> [_ w191 w225]
          tunnel: w163 -> [_ w190 w224]
          tunnel: w162 -> [_ w189 w226]
          tunnel: [w175 w186 w226] -> w140
          tunnel: [w176 w187 w224] -> w141
          tunnel: [w177 w188 w225] -> w142
          tunnel: w160 -> [_ w192 _]
          tunnel: w139 -> [_ w182 _]
          tunnel: w138 -> [_ w181 _]
          tunnel: [w174 w179 w223] -> w133
          tunnel: w137 -> [w174 w180 w223]
          frame "Sub Cooled", Default {
          }
          frame "Saturation" {
            n253 = case shown="\"4\"" w192 {
              tunnel: w191 -> [_ w201 w205 _ _]
              tunnel: w190 -> [_ w200 w204 _ _]
              tunnel: w189 -> [_ w199 w203 _ _]
              tunnel: [0.0 ("S") w201 w205 w209 w212] -> w188
              tunnel: [0.0 ("H Point 3") w200 w204 w207 w211] -> w187
              tunnel: [0.0 ("V") w199 w203 w208 w210] -> w186
              tunnel: w185 -> [_ _ _ w209 _]
              tunnel: w184 -> [_ _ _ w207 _]
              tunnel: w183 -> [_ _ _ w208 _]
              tunnel: w182 -> [_ _ _ _ w222]
              tunnel: w181 -> [_ _ _ _ w214]
              tunnel: w180 -> [_ w198 w202 w206 _]
              tunnel: [0.0 ("V") w198 w202 w206 w213] -> w179
              frame "0" {
                # "No Thing"
              }
              frame "1" {
                # "Saturated Vapor"
              }
              frame "2" {
                # "Saturated Vapor"
              }
              frame "3" {
                # "Sub Cooled"
                n254 = local write "H Point 3"(w207) -> ()
              }
              frame "4" {
                n255 = Unbundle By Name(w214) -> ("H"=w220:dbl, "H 2"=w219:dbl)
                n256 = Unbundle By Name(w214) -> ("S"=w218:dbl, "S 2"=w217:dbl, "V"=w216:dbl, "V 2"=w215:dbl)
                n257 = Unbundle By Name(w222) -> ("H"=w221:dbl)
                n258 = formula code="float64 x;\nfloat64 v;\nfloat64 s;\n\nx = (h-h1)/(h2-h1);\ns = s1 + x*(s2-s1);\nv = v1 + x*(v2-v1);"("h"=w221, "h1"=w220, "h2"=w219, "s1"=w218, "s2"=w217, "v1"=w216, "v2"=w215) -> ("x"=w213:dbl, "s"=w212:dbl, "h"=w211:dbl, "v"=w210:dbl)
              }
            }
          }
          frame "Super Heated" {
          }
        }
        n259 = Increment(x=w149) -> (x+1=w145:i32)
        n260 = Number To Fractional String(number=w143, precision (6)=i16 3) -> (F-format string=w153:string)  [unwired: 2 in]
        n261 = Number To Fractional String(number=w144, precision (6)=i16 3 ("width (-)")) -> (F-format string=w151:string)  [unwired: 2 in]
        n262 = Number To Decimal String(number=w145, width (-)=i16 3) -> (decimal integer string=w168:string)
        n263 = Number To Fractional String(number=w142, precision (6)=i16 3) -> (F-format string=w156:string)  [unwired: 2 in]
        n264 = Number To Fractional String(number=w141, precision (6)=i16 3) -> (F-format string=w158:string)  [unwired: 2 in]
        n265 = Number To Fractional String(number=w140, precision (6)=i16 3) -> (F-format string=w154:string)  [unwired: 2 in]
        n266 = Number To Fractional String(number=w133, precision (6)=i16 3) -> (F-format string=w135:string)  [unwired: 2 in]
        n267 = Build Array(w145, w144, w143, w142, w141, w140, 0.0 ("element"), w133) -> (w146:dbl[])
        n268 = Build Array(w168, w151, w153, w156, w158, w154, w161, w135) -> (w173:string[])
        n269 = Insert Into Array(array=w172, new element=w173) -> (w171:string[][])  [unwired: 2 in]
        n270 = Insert Into Array(array=w147, new element=w146) -> (w148:dbl[][])  [unwired: 2 in]
        "Loop Iteration" <- w149
      }
      "Table" <- w59
      "Points" <- w48
      n271 = Index Array(array=w59, index (col)=4 ("disabled index (col)")) -> (element=w60:string[])  [unwired: 1 in]
      n272 = Index Array(array=w59, index (col)=2 ("disabled index (col)")) -> (element=w61:string[])  [unwired: 1 in]
      n273 = for {
        tunnel: w60 -> [w127] mode=indexing
        tunnel: w61 -> [w126] mode=indexing
        shift-right: [w130] -> w62
        shift-left: dbl[] [] -> [w132]
        shift-right: [w129] -> w63
        shift-left: dbl[] [] -> [w131]
        i -> [w128]
        n274 = Fract/Exp String To Number(string=w127) -> (number=w125:dbl)  [unwired: 3 in, 1 out]
        n275 = Fract/Exp String To Number(string=w126) -> (number=w124:dbl)  [unwired: 3 in, 1 out]
        n276 = Insert Into Array(array=w132, index=w128, new element=w125) -> (w130:dbl[])
        n277 = Insert Into Array(array=w131, index=w128, new element=w124) -> (w129:dbl[])
      }
      n278 = Bundle(w62, w63) -> (w50:cluster{dbl[], dbl[]})  [unwired: 1 in]
      "output cluster" <- w50
      "XY Graph" <- w50
      n279 = call "Initialize_Graph.vi"("XYGraph in"="XY Graph Ref In") -> ("error out"=w51:errorcluster)  [unwired: 10 in]
      n280 = property class="XYGraph (strict)"(reference="XY Graph Ref In", error in=w51) -> (reference out=w64:refnum<vi>, error out=w65:errorcluster, "Value"=w42:cluster{"all rows":dbl[], "all rows":dbl[]}[])
      n281 = Build Array (concatenate)(w42, w50) -> (w46:cluster{"all rows":dbl[], "all rows":dbl[]}[])
      n282 = local read "Cycle"() -> (w33:string)
      n283 = property class="XYGraph (strict)"(reference=w64, error in=w65, "Val(Sgnl)"=w46, "Visible"=TRUE) -> (reference out=w47:refnum<vi>)  [unwired: 1 out]
      n284 = Array Size(array=w46) -> (size(s)=w45:i32)
      n285 = Decrement(x=w45) -> (x-1=w32:i32)
      n286 = case shown="\"Cycle 4\"" w33 {
        tunnel: [string[] ["1,6", "2", "3,4", "5"] string[] ["1,6", "2", "3", "4", "5"] string[] ["1,6", "2", "3", "4", "5"] string[] ["1,9", "2", "3,7", "8"] string[] ["1,9", "2", "3", "7", "8"] string[] ["1,9", "2", "3", "7", "8"] string[] ["1", "2", "3,4,7", "8", "9", "5", "6"] string[] ["1", "2", "3", "7", "8", "9", "4", "5", "6"] string[] ["1", "2", "3", "7", "8", "9", "4", "5", "6"]] -> w35
        tunnel: [i32[] [0, 2, 3, 5] i32[] [0, 2, 3, 4, 5] i32[] [0, 2, 3, 4, 5] i32[] [0, 2, 3, 5] i32[] [0, 2, 3, 4, 5] i32[] [0, 2, 3, 4, 5] i32[] [0, 1, 2, 4, 5, 10, 11] i32[] [0, 1, 2, 3, 4, 5, 9, 10, 11] i32[] [0, 1, 2, 3, 4, 5, 9, 10, 11]] -> w34
        frame "Cycle 1", Default {
        }
        frame "Cycle 2" {
        }
        frame "Cycle 3" {
        }
        frame "Cycle 4" {
        }
        frame "Cycle 5" {
        }
        frame "Cycle 6" {
        }
        frame "Cycle 7" {
        }
        frame "Cycle 8" {
        }
        frame "Cycle 9" {
        }
      }
      n287 = property class="XYGraph (strict)"(reference=w47, "Active Plot"=w32, "Plot.Line Width"=5, "Plot.Plot Color"=u32 0) -> (reference out=w27:refnum<vi>, error out=w26:errorcluster)  [unwired: 1 in]
      n288 = property on="Property Node" class="XYGraph (strict)"(reference=w27, error in=w26) -> (reference out=w38:refnum<vi>, error out=w37:errorcluster, "AnntList"=w40:T7)
      n289 = for {
        tunnel: w41 -> [w110]
        shift-right: [w108] -> w39
        shift-left: w40 -> [w107]
        tunnel: w35 -> [w106] mode=indexing
        tunnel: w34 -> [w105] mode=indexing
        tunnel: w32 -> [w104]
        n290 = Bundle By Name(cluster=w110, "Name"=w106, "Color"=u32 0, "Style"=u8 0, "Point Style"=u8 0, "Name Visible"=TRUE, "Allow Drag"=FALSE, "Annotation Mode"=u32 1, "Plot"=w104, "Index"=w105, "Position"=cluster{"X":dbl, "Y":dbl} {"X"=1.0, "Y"=1.0}, "X Scale"=u32 0, "Y Scale"=u32 0, "Show Arrow"=FALSE, "Lock Name"=TRUE, "Plot Area"=0, "Label Offset"=cluster{"X":dbl, "Y":dbl} {"X"=10.0, "Y"=0.5}) -> (w109:T4)
        n291 = Build Array (concatenate)(w107, w109) -> (w108:T7)
      }
      n292 = property on="Property Node" class="XYGraph (strict)"(reference=w38, error in=w37, "AnntList"=w39) -> (reference out=w31:refnum<vi>, error out=w30:errorcluster)
      n293 = invoke class="XYGraph (strict)" method="ForceRedraw"(reference=w31, error in=w30) -> (reference out=w29:refnum<vi>, error out=w28:errorcluster)  [unwired: 1 in, 1 out]
      n294 = disable-structure shown="Disabled" {
        disable-tunnel: w29 -> [w83 w85]
        disable-tunnel: w28 -> [w82 w84]
        disable-tunnel: [w70 w85] -> w25
        disable-tunnel: [w69 w84] -> w24
        frame Disabled {
          # "Exporting Graph into image"
          n295 = call <vilib>:"Application Directory.vi"() -> ("Application Directory"=w72:path)
          "Application Directory 2" <- w72
          n296 = Build Path(base path=w72, name or relative path="Cycles_Images") -> (appended path=w68:path)
          n297 = Create Folder(path (use dialog)=w68) -> (created path=w67:path, error out=→"error out":errorcluster)  [unwired: 2 in, 1 out]
          n298 = Format Date/Time String(time format string (%c)=" %d%m%y_%H%M") -> (date/time string=w73:string)  [unwired: 2 in]
          n299 = Concatenate Strings("image_" ("name or relative path"), w73) -> (w75:string)
          n300 = Build Path(base path=w67, name or relative path=w75) -> (appended path=w77:path)
          "Application Directory" <- w77
          n301 = invoke class="XYGraph (strict)" method="Export Image"(reference=w83, error in=w82, "FileType"=enum32{"BMP", "EPS", "EMF", "PICT"}."BMP" ("File Type"), "Target"=enum32{"File", "Clipboard"}."File", "Path"=w77, "HideGrid"=TRUE ("Hide Grid"), "Overwrite"=TRUE ("Always Overwrite")) -> (reference out=w70:refnum<vi>, error out=w69:errorcluster)  [unwired: 1 in, 6 out]
        }
        frame Enabled {
        }
      }
      "XY Graph Ref Out" <- w25
      n302 = call <vilib>:"Simple Error Handler.vi"("error in (no error)"=w24) -> ()  [unwired: 4 in, 5 out]
    }
  }
